vi "Write Setup.vi"(8 "error in (no error)":errorcluster, 11 "Channel in":refnum<class "Channel.lvclass">) -> (0 "error out":errorcluster, 3 "Channel out":refnum<class "Channel.lvclass">)   [LabVIEW 2018, in "Channel.lvclass"]
uses:
  Channel.lvclass
  Channel.lvclass/Channel.ctl
  Interface/Interface.lvclass
  RxTx/RxTx.lvclass
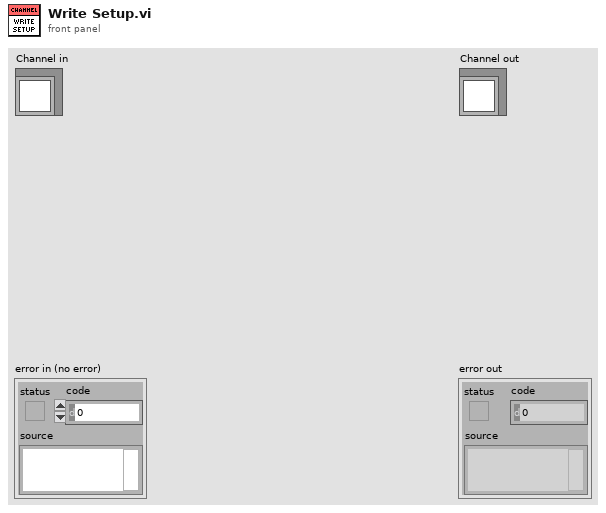
[diagram p1: front panel]
types:
  T1 = cluster{"Exposure Time":sgl, "Pre-amp gain":u8, "Readout Rate":u8, "EM Mode":u8, "EM Gain":u16, "Binning":u16, "Initial Line":u16, "Initial Cloumn":u16, "Final Line":u16, "Final Column":u16, "Kinetic Series Length":u32, "Shutter Mode":u8, "Cooler ON/OFF":u16, "Temperature":i8, "Image Name":string, "Image Path":string, "Cubes":u32, "Trigger":u16}
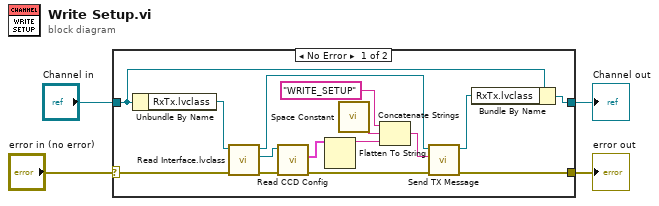
[diagram p0: block diagram]
diagram:
  n1 = case shown="No Error" "error in (no error)" {
    selector: "error in (no error)" -> [w19 w21]
    tunnel: [w5 w21] -> w3
    tunnel: [w6 w20] -> w1
    tunnel: "Channel in" -> [w7 w20]
    frame No Error {
      n2 = Unbundle By Name(w7) -> ("RxTx.lvclass"=w18:refnum<class "RxTx.lvclass">)
      n3 = call "Read Interface.lvclass.vi"("error in (no error)"=w19, "RxTx in"=w18) -> ("error out"=w16:errorcluster, "Interface.lvclass"=w17:refnum<class "Interface.lvclass">, "RxTx out"=w10:refnum<class "RxTx.lvclass">)  [unwired: 7 in]
      n4 = call "Read CCD Config.vi"("error in (no error)"=w16, "Interface in"=w17) -> ("error out"=w9:errorcluster, "CCD Config"=w15:T1)  [unwired: 7 in, 1 out]
      n5 = Flatten To String(anything=w15) -> (data string=w13:string)  [unwired: 3 in, 2 out]
      n6 = call <vilib>:"Space Constant.vi"() -> ("String"=w12:string)
      n7 = Concatenate Strings("WRITE_SETUP" ("string"), w12, w13) -> (w11:string)
      n8 = call "Send TX Message.vi"("error in (no error)"=w9, "message"=w11, "RxTx in"=w10) -> ("error out"=w5:errorcluster, "RxTx out"=w8:refnum<class "RxTx.lvclass">)  [unwired: 7 in]
      n9 = Bundle By Name(cluster=w7, "RxTx.lvclass"=w8) -> (w6:refnum<class "Channel.lvclass">)
    }
    frame Error {
    }
  }
  "error out" <- w3
  "Channel out" <- w1
